vi "loadDataNodeEnd.vi"(8 "error in (no error)":errorcluster, 10 "XML Refnum in":refnum<file>, 11 "xceDataNode in":refnum<class "xceDataNode.lvclass">) -> (0 "error out":errorcluster, 2 "XML Refnum out":refnum<file>, 3 "xceDataNode out":refnum<class "xceDataNode.lvclass">)   [LabVIEW 2013, in "xceDataNode.lvclass"]
doc: "Part of the file loading process. Occurs at the end of a node being loaded. Includes checking the end of the tag which has the format </tag>."
uses:
  xceDataNode.lvclass
  xceNode/xceNode.lvclass
  XML Parser/XML Parser.lvclass
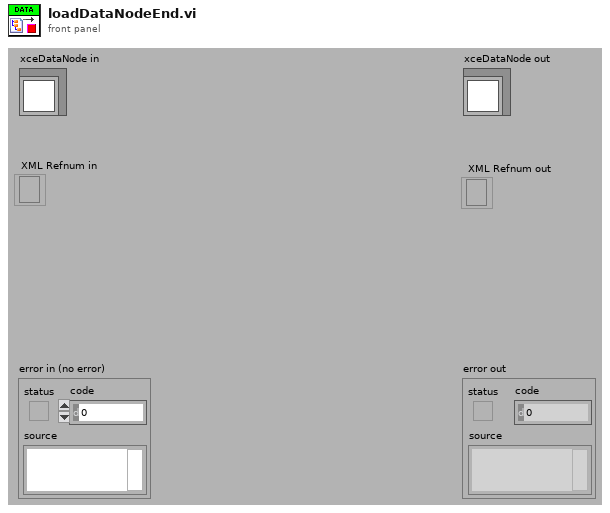
[diagram p1: front panel]
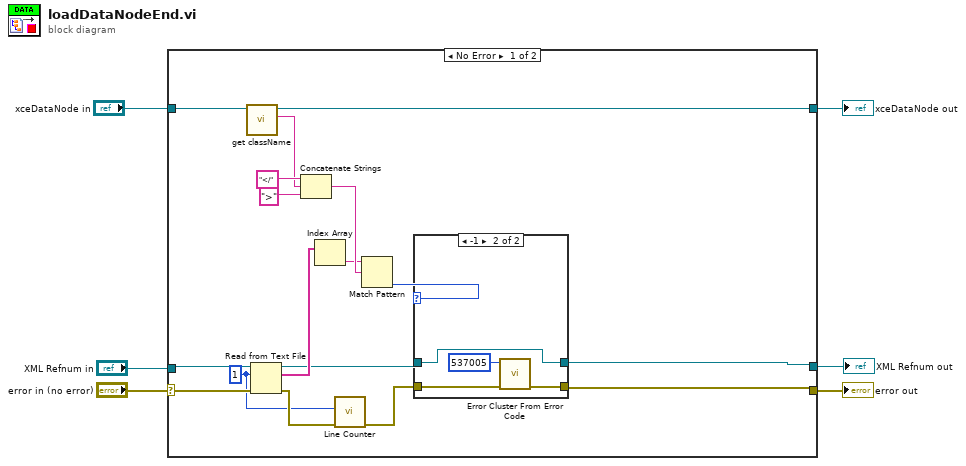
[diagram p0: block diagram]
diagram:
  n1 = case shown="No Error" "error in (no error)" {
    selector: "error in (no error)" -> [w23 w32]
    tunnel: [w11 w32] -> w5
    tunnel: [w20 w31] -> w3
    tunnel: "xceDataNode in" -> [w21 w31]
    tunnel: "XML Refnum in" -> [w22 w30]
    tunnel: [w10 w30] -> w1
    frame No Error {
      w7 = 1 ("count")
      n2 = call "get className.vi"("xceNode in"=w21) -> ("Class name"=w18:string, "xceNode out"=w20:refnum<class "xceDataNode.lvclass">)  [unwired: 8 in, 1 out]
      n3 = Read from Text File(file (use dialog)=w22, count=w7, error in=w23) -> (refnum out=w12:refnum<file>, text=w15:string[], error out=w9:errorcluster)  [unwired: 1 in, 1 out]
      n4 = Concatenate Strings("</", w18, ">") -> (w16:string)
      n5 = Index Array(array=w15) -> (element=w14:string)  [unwired: 1 in]
      n6 = call "Line Counter.vi"("error in (no error)"=w9, "# of lines to increment (1)"=w7) -> ("error out"=w8:errorcluster)  [unwired: 8 in, 1 out]
      n7 = Match Pattern(string=w14, regular expression=w16) -> (offset past match=w13:i32)  [unwired: 1 in, 3 out]
      n8 = case shown="-1" w13 {
        tunnel: w8 -> [w25 w29]
        tunnel: [w25 w27] -> w11
        tunnel: w12 -> [w24 w26]
        tunnel: [w24 w26] -> w10
        frame 0, Default {
        }
        frame -1 {
          n9 = call <vilib>:"Error Cluster From Error Code.vi"("error in (no error)"=w29, "error code (0)"=537005) -> ("error out"=w27:errorcluster)  [unwired: 7 in]
        }
      }
    }
    frame Error {
    }
  }
  "error out" <- w5
  "xceDataNode out" <- w3
  "XML Refnum out" <- w1
